vi "BallSequencing.vi"(0 "Balls In Robot":i32, 1 "Speed of Harvester":dbl, 5 "Shoot":bool, 7 "Ball S12 Process":bool, 9 "Ball S3 Process":bool, 11 "Speed of Conveyor":dbl, 12 "SP 1 Triggered":bool, 13 "SP 2 Triggered":bool, 14 "SP 3 Triggered":bool) -> (2 "Conveyer Output":dbl, 3 "Harvester Output":dbl, 4 "Balls In Robot Output":i32, 6 "Shoot Output":bool, 8 "Ball S12 Process Output":bool, 10 "Ball S3 Process Output":bool)   [LabVIEW 2011]
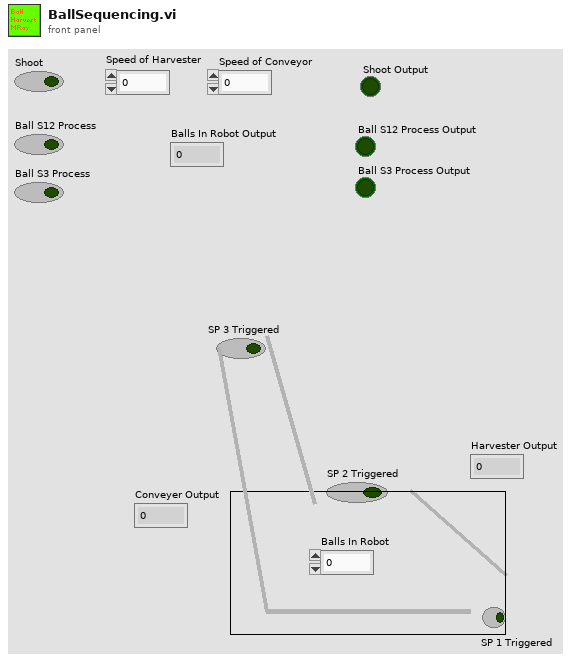
[diagram p1: front panel]
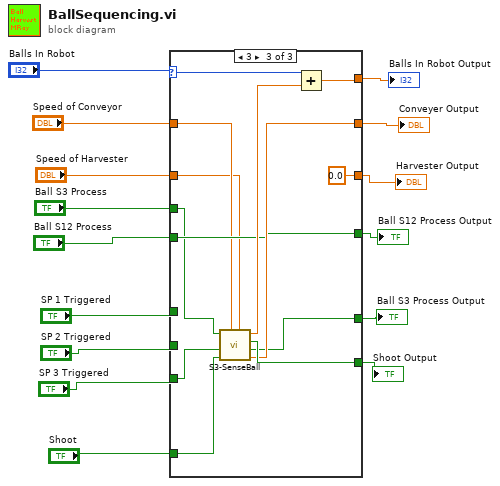
[diagram p0: block diagram]
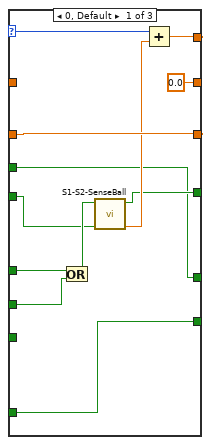
[diagram p2: hidden frame]
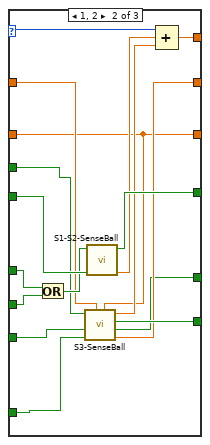
[diagram p3: hidden frame]
diagram:
  n1 = case shown="3" "Balls In Robot" {
    selector: "Balls In Robot" -> [w26 w37 w56]
    tunnel: "SP 1 Triggered" -> [w23 w42 _]
    tunnel: "SP 2 Triggered" -> [w22 w43 _]
    tunnel: [w27 w28 0.0 ("Speed of Harvester")] -> w15
    tunnel: "Speed of Harvester" -> [w27 w28 w47]
    tunnel: "Speed of Conveyor" -> [_ w29 w48]
    tunnel: [0.0 ("Conveyer Output") w31 w50] -> w3
    tunnel: [w25 w39 w55] -> w2
    tunnel: "SP 3 Triggered" -> [_ w35 w51]
    tunnel: "Ball S3 Process" -> [w17 w34 w46]
    tunnel: "Ball S12 Process" -> [w20 w44 w49]
    tunnel: [w19 w40 w49] -> w4
    tunnel: "Shoot" -> [w18 w36 w54]
    tunnel: [w18 w33 w53] -> w5
    tunnel: [w17 w30 w45] -> w1
    frame 0, Default {
      n2 = Or(x=w23, y=w22) -> (x .or. y?=w21:bool)
      n3 = call "S1-S2-SenseBall.vi"("Ball in Process in"=w20, "Sense Ball"=w21) -> ("Ball Counter"=w24:dbl, "Ball in Process out"=w19:bool)  [unwired: 8 in]
      n4 = Add(x=w26, y=w24) -> (x+y=w25:dbl)
    }
    frame 1, 2 {
      n5 = Or(x=w42, y=w43) -> (x .or. y?=w41:bool)
      n6 = call "S3-SenseBall.vi"("Harvester Speed"=w28, "Conveyor Speed"=w29, "Shoot"=w36, "Sense Ball"=w35, "Ball S3 Process"=w34) -> ("Conveyer Output"=w31:dbl, "Ball S3 Process Output"=w30:bool, "Shoot Output"=w33:bool, "Ball Counter"=w32:dbl)  [unwired: 3 in]
      n7 = call "S1-S2-SenseBall.vi"("Ball in Process in"=w44, "Sense Ball"=w41) -> ("Ball Counter"=w38:dbl, "Ball in Process out"=w40:bool)  [unwired: 8 in]
      n8 = Compound Arithmetic op=ADD(w37, w38, w32) -> (w39:dbl)
    }
    frame 3 {
      n9 = call "S3-SenseBall.vi"("Harvester Speed"=w47, "Conveyor Speed"=w48, "Shoot"=w54, "Sense Ball"=w51, "Ball S3 Process"=w46) -> ("Conveyer Output"=w50:dbl, "Ball S3 Process Output"=w45:bool, "Shoot Output"=w53:bool, "Ball Counter"=w52:dbl)  [unwired: 3 in]
      n10 = Add(x=w56, y=w52) -> (x+y=w55:dbl)
    }
  }
  "Shoot Output" <- w5
  "Ball S12 Process Output" <- w4
  "Harvester Output" <- w15
  "Conveyer Output" <- w3
  "Balls In Robot Output" <- w2
  "Ball S3 Process Output" <- w1
